vi "Search IO Devices.vi"(11 "Host Resources":T1) -> (0 "By Slot":i32[](array[numeric]), 1 "By Product Name":string[](array[string]), 2 "By Model Number":u32[](array[numeric]), 3 "By Alias":string[](array[string]))   [LabVIEW 2021, in "Load Frame.lvlib"]
uses:
  Load Frame.lvlib
  Acquisition/Host Resources.ctl
  Acquisition/Host Software Package.ctl
  Acquisition/Host IO Resource.ctl
  Acquisition/Acquisition.lvlib
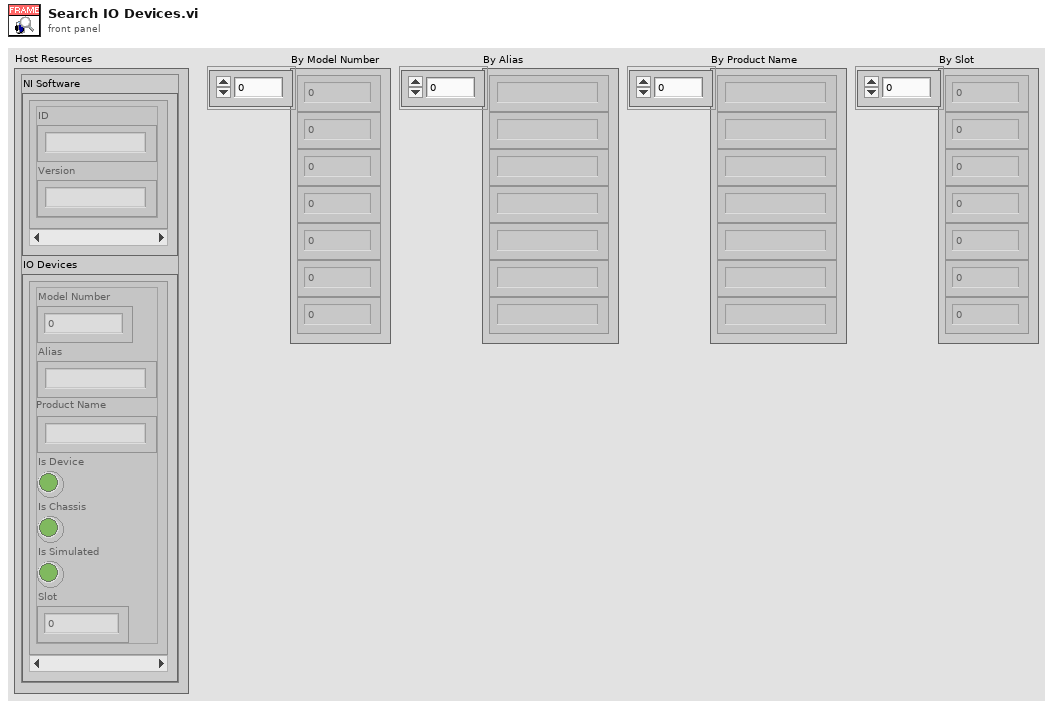
[diagram p1: front panel]
types:
  T1 = typedef "Acquisition.lvlib/Host Resources.ctl" = cluster{"NI Software":T2[], "IO Devices":T3[]}
  T2 = typedef "Acquisition.lvlib/Host Software Package.ctl" = cluster{"ID":string, "Version":string}
  T3 = typedef "Acquisition.lvlib/Host IO Resource.ctl" = cluster{"Model Number":u32, "Alias":string, "Product Name":string, "Is Device":bool, "Is Chassis":bool, "Is Simulated":bool, "Slot":i32}
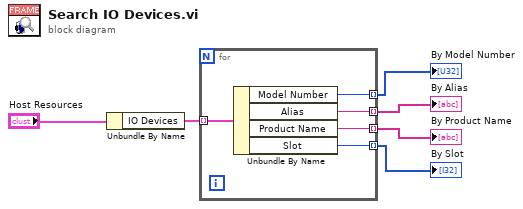
[diagram p0: block diagram]
diagram:
  n1 = Unbundle By Name("Host Resources") -> ("IO Devices"=w6:T3[])
  n2 = for {
    tunnel: w6 -> [w11] mode=indexing
    tunnel: [w10] -> w4 mode=indexing
    tunnel: [w9] -> w3 mode=indexing
    tunnel: [w8] -> w2 mode=indexing
    tunnel: [w7] -> w1 mode=indexing
    n3 = Unbundle By Name(w11) -> ("Model Number"=w10:u32, "Alias"=w9:string, "Product Name"=w8:string, "Slot"=w7:i32)
  }
  "By Model Number" <- w4
  "By Alias" <- w3
  "By Product Name" <- w2
  "By Slot" <- w1
